vi "Quad.vi"(2 "Chaotic parameter":dbl=3.4 format="%.2f", 3 "Number of Iterates to compute":dbl=25.0 format="%.2f", 4 "Number of pre-iterates":dbl=300.0 format="%.2f", 5 "Initial Value":dbl=0.01 format="%.2f") -> (0 "Array of Xn":dbl[](graph)=[0.03366, 0.11059181496, 0.3344283024411006, 0.7567924440893788, 0.625795978239251, 0.7961962643200216, 0.5517104282097374, 0.840908507488843, 0.4548567243738801, 0.84307108786353, 0.4498275774852558, 0.8414412752646068, 0.45362070885530864, 0.8426864685999144, 0.4507243464109677, 0.8417444938754705, 0.452916383079715, 0.8424626522601931, 0.4512457281435077, 0.841918271317527, 0.4525124455133957, 0.8423327693741979, 0.4515481350428136, 0.8420182170593798, 0.45228003327837796], 1 "Final iterate":dbl=0.45228003327837796 format="%.2f")   [LabVIEW 2012]
doc: "iterates the quadratic map, returning an array of N iterates after pre-iterating the specified number of times."
panel:
  # "Time-series data from the quadratic map"
  # "Xn"
  # "Iterate #"
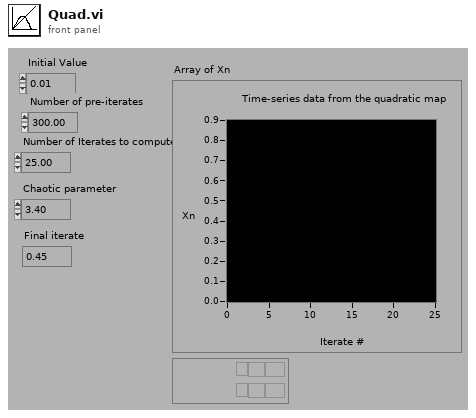
[diagram p1: front panel]
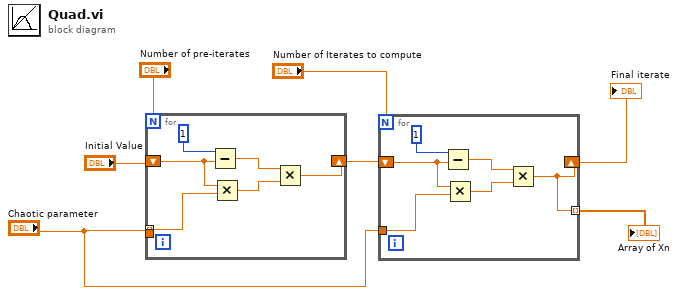
[diagram p0: block diagram]
diagram:
  n1 = for {
    N: "Number of pre-iterates" -> [_]
    shift-right: [w9] -> w2
    shift-left: "Initial Value" -> [w12]
    tunnel: [w8] -> _ mode=indexing
    tunnel: "Chaotic parameter" -> [w8]
    n2 = Subtract(x=1, y=w12) -> (x-y=w10:dbl)
    n3 = Multiply(x=w12, y=w8) -> (x*y=w11:dbl)
    n4 = Multiply(x=w10, y=w11) -> (x*y=w9:dbl)
  }
  n5 = for {
    N: "Number of Iterates to compute" -> [_]
    shift-right: [w14] -> w6
    shift-left: w2 -> [w18]
    tunnel: "Chaotic parameter" -> [w15]
    tunnel: [w14] -> w5 mode=indexing
    n6 = Subtract(x=1, y=w18) -> (x-y=w16:dbl)
    n7 = Multiply(x=w18, y=w15) -> (x*y=w17:dbl)
    n8 = Multiply(x=w16, y=w17) -> (x*y=w14:dbl)
  }
  "Array of Xn" <- w5
  "Final iterate" <- w6
